vi "radio_test.vi"() -> ()   [LabVIEW 2019]
uses:
  Radio_Speed_Ctrl.ctl
panel:
  out "Speed":dbl
  out "Raw":dbl
  out "Left Speed \nDemand\nPERCENT":T1=enum."Radio Selection 7"
  in  "Left Speed \nDemand\nPERCENT":T1=enum."Radio Selection 7"
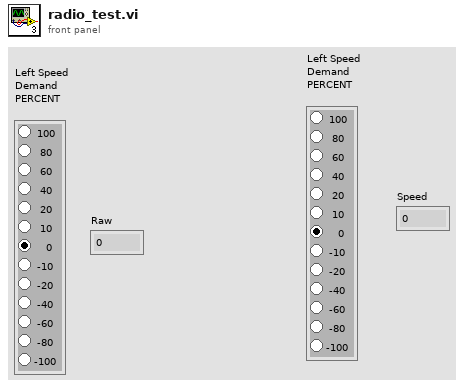
[diagram p1: front panel]
types:
  T1 = typedef "Radio_Speed_Ctrl.ctl" = enum32{"Radio Selection 1", "Radio Selection 2", "Radio Selection 3", "Radio Selection 4", "Radio Selection 5", "Radio Selection 6", "Radio Selection 7", "Radio Selection 8", "Radio Selection 9", "Radio Selection 10", "Radio Selection 11", "Radio Selection 12", "Radio Selection 13"}
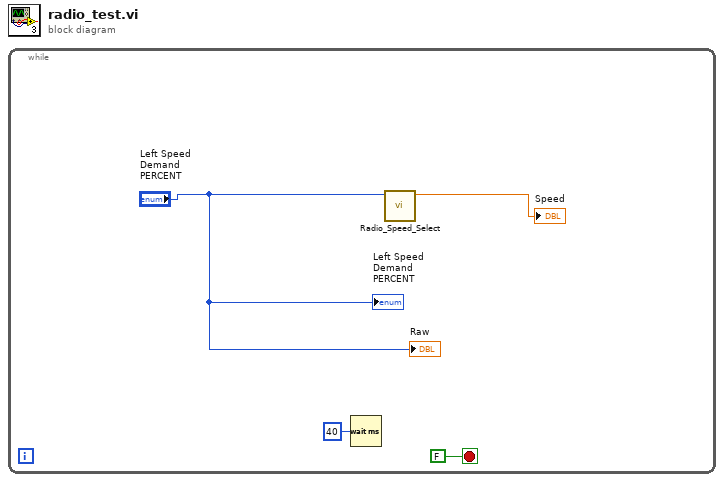
[diagram p0: block diagram]
diagram:
  n1 = while {
    stop <- FALSE stop-if-true
    n2 = Wait (ms)(milliseconds to wait=u32 40) -> ()  [unwired: 1 out]
    n3 = call "Radio_Speed_Select.vi"("Left Speed \nDemand\nPERCENT"="Left Speed \nDemand\nPERCENT") -> ("PERCENT"=→"Speed":dbl)  [unwired: 10 in]
    "Left Speed \nDemand\nPERCENT" <- "Left Speed \nDemand\nPERCENT"
    "Raw" <- "Left Speed \nDemand\nPERCENT"
  }
